vi "Format TCS String.vi"(8 "error in (no error)":errorcluster, 10 "String in":string, 11 "S4GUI in":refnum<class "S4GUI.lvclass">) -> (0 "error out":errorcluster, 2 "String out":string, 3 "S4GUI out":refnum<class "S4GUI.lvclass">)   [LabVIEW 2018]
uses:
  S4GUI.lvclass
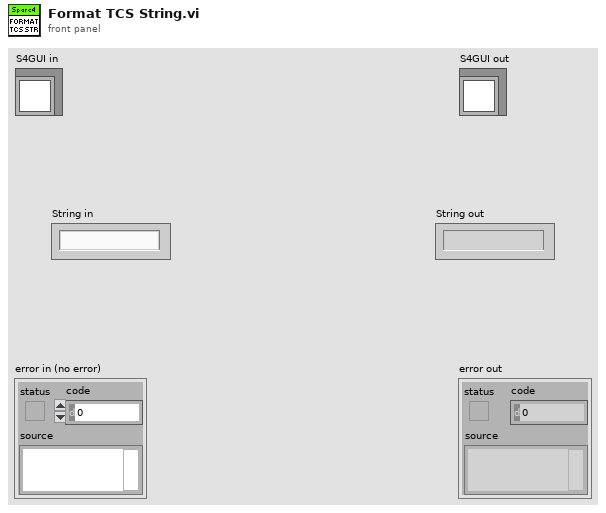
[diagram p1: front panel]
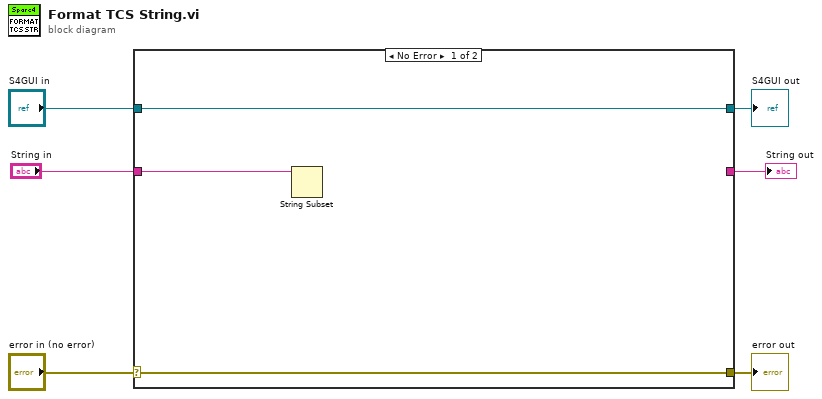
[diagram p0: block diagram]
diagram:
  n1 = case shown="No Error" "error in (no error)" {
    selector: "error in (no error)" -> [w8 w12]
    tunnel: [w8 w12] -> w5
    tunnel: [w9 w11] -> w3
    tunnel: "S4GUI in" -> [w9 w11]
    tunnel: "String in" -> [w7 w10]
    tunnel: [_ w10] -> w1
    frame No Error {
      n2 = String Subset(string=w7) -> ()  [unwired: 2 in, 1 out]
    }
    frame Error {
    }
  }
  "error out" <- w5
  "S4GUI out" <- w3
  "String out" <- w1
